vi "CAN2MsgList.vi"(0 "Direction":bool, 1 "VCI_CAN_OBJ":T1={"ID"=0, "TimeStamp"=0, "TimeFlag"=0, "SendType"=1, "RemoteFlag"=0, "ExternFlag"=0, "DataLen"=8, "Data0"=0, "Data1"=0, "Data2"=0, "Data3"=0, "Data4"=0, "Data5"=0, "Data6"=0, "Data7"=0, "Reserved"=0, 0, 0}) -> (3 "CAN Message":string[](array[string]))   [LabVIEW 2017]
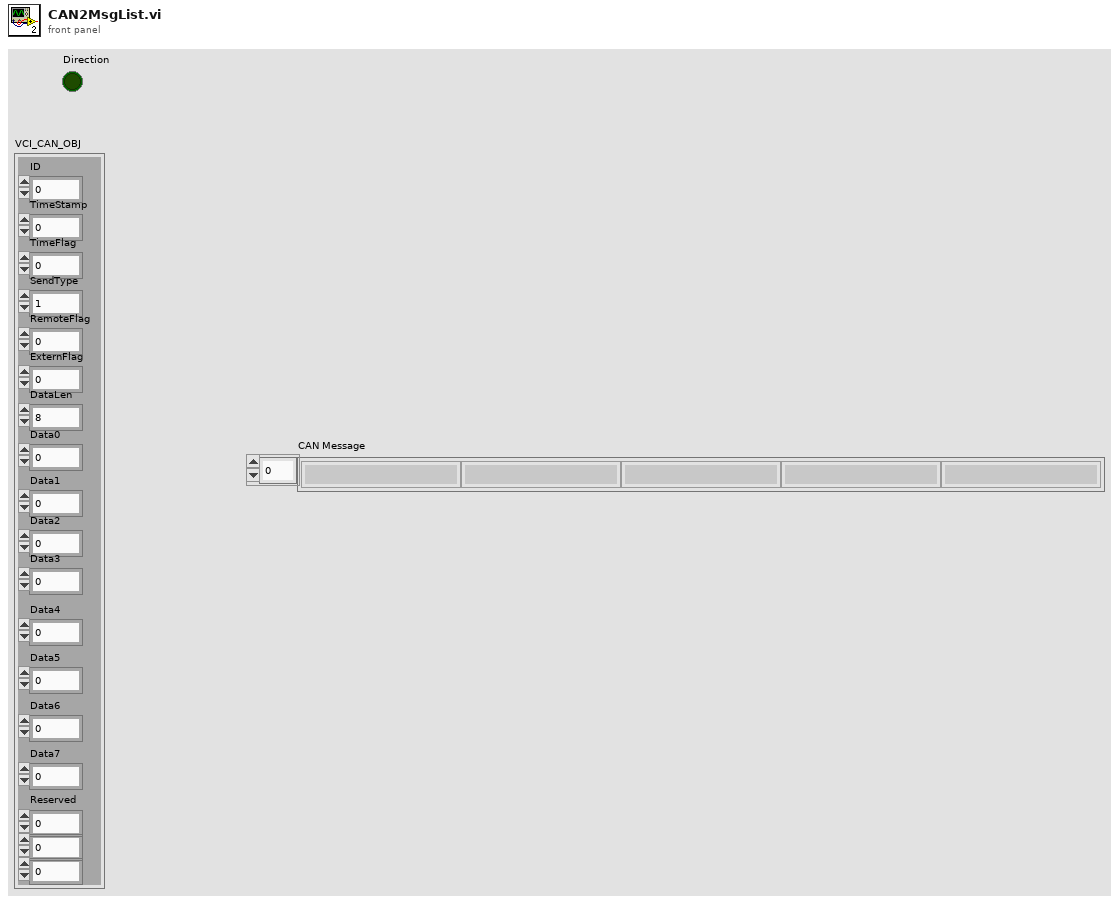
[diagram p1: front panel]
types:
  T1 = cluster{"ID":u32, "TimeStamp":u32, "TimeFlag":u8, "SendType":u8, "RemoteFlag":u8, "ExternFlag":u8, "DataLen":u8, "Data0":u8, "Data1":u8, "Data2":u8, "Data3":u8, "Data4":u8, "Data5":u8, "Data6":u8, "Data7":u8, "Reserved":u8, u8, u8}
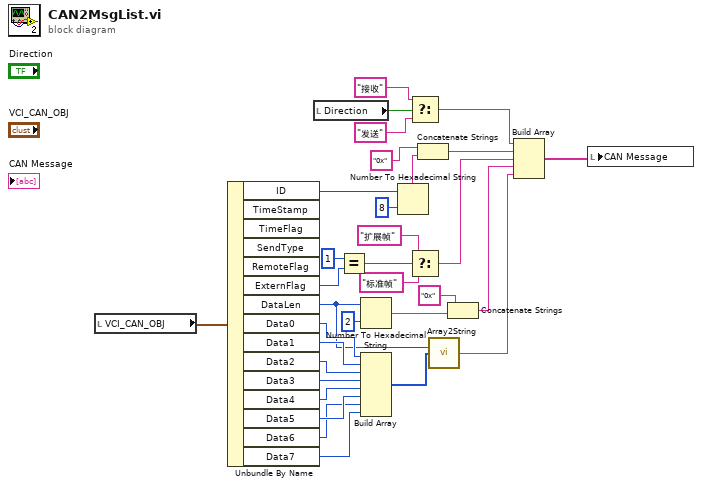
[diagram p0: block diagram]
diagram:
  n1 = local read "VCI_CAN_OBJ"() -> (w28:T1)
  n2 = Unbundle By Name(w28) -> ("ID"=w26:u32, "ExternFlag"=w14:u8, "DataLen"=w1:u8, "Data0"=w12:u8, "Data1"=w11:u8, "Data2"=w10:u8, "Data3"=w9:u8, "Data4"=w8:u8, "Data5"=w7:u8, "Data6"=w6:u8, "Data7"=w5:u8)  [unwired: 4 out]
  n3 = local read "Direction"() -> (w32:bool)
  n4 = Equal?(x=u8 1, y=w14) -> (x = y?=w25:bool)
  n5 = Number To Hexadecimal String(1:i16 2 ("宽度(-)"), 2:w1) -> (0:w20:string)
  n6 = Build Array(w12, w11, w10, w9, w8, w7, w6, w5) -> (w2:u8[])
  n7 = Number To Hexadecimal String(1:i16 8 ("宽度(-)"), 2:w26) -> (0:w17:string)
  n8 = Select(t="接收", s=w32, f="发送") -> (s? t:f=w31:string)
  n9 = Select(t="扩展帧", s=w25, f="标准帧") -> (s? t:f=w22:string)
  n10 = Concatenate Strings("0x" ("字符串"), w17) -> (w15:string)
  n11 = call "Array2String.vi"("Size"=w1, "Hex Array"=w2) -> ("HEX String"=w3:string)  [unwired: 13 in]
  n12 = Concatenate Strings("0x" ("字符串"), w20) -> (w18:string)
  n13 = Build Array(w31, w15, w22, w18, w3) -> (w4:string[])
  n14 = local write "CAN Message"(w4) -> ()
